vi "Set Window Title.vi"(8 "error in (no error)":errorcluster, 10 "Window Title":string, 11 "VI Refnum In":refnum<vi>) -> (0 "error out":errorcluster, 3 "VI Refnum Out":refnum<vi>)   [LabVIEW 2019, in "UI Tools.lvlib"]
doc: "Set Window Titel."
uses:
  UI Tools.lvlib
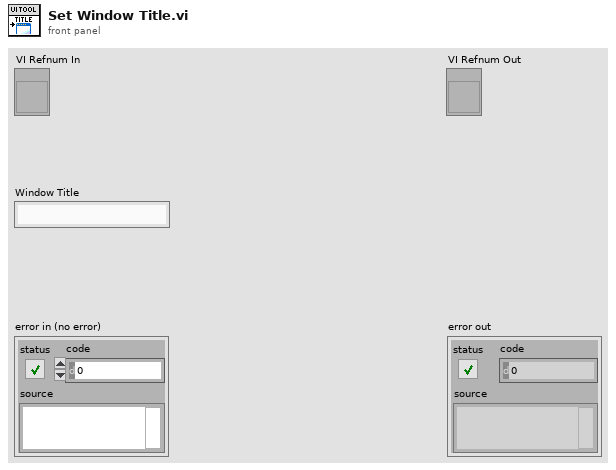
[diagram p1: front panel]
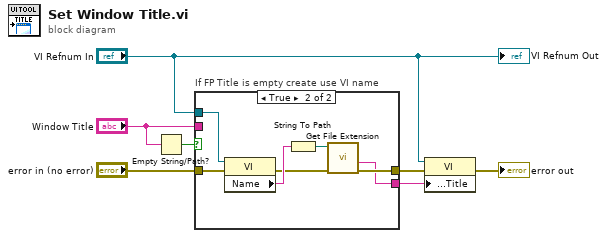
[diagram p0: block diagram]
diagram:
  n1 = Empty String/Path?(string/path="Window Title") -> (empty?=w7:bool)
  n2 = case "If FP Title is empty create use VI name" shown="True" w7 {
    tunnel: "Window Title" -> [w8 _]
    tunnel: "error in (no error)" -> [w9 w13]
    tunnel: [w9 w12] -> w4
    tunnel: [w8 w11] -> w5
    tunnel: "VI Refnum In" -> [_ w10]
    frame False {
    }
    frame True {
      n3 = property class="VI"(reference=w10, error in=w13) -> (error out=w14:errorcluster, "Name"=w16:string)  [unwired: 1 out]
      n4 = String To Path(string=w16) -> (path=w15:path)
      n5 = call <vilib>:"Get File Extension.vi"("error in (no error)"=w14, "file"=w15) -> ("error out"=w12:errorcluster, "filename without extension"=w11:string)  [unwired: 8 out]
    }
  }
  n6 = property class="VI"(reference="VI Refnum In", error in=w4, "Front Panel.Title"=w5) -> (error out=→"error out":errorcluster)  [unwired: 1 out]
  "VI Refnum Out" <- "VI Refnum In"
